vi "Reference Example.vi"() -> ()   [LabVIEW 2016, in "CS++Core-Examples.lvlib"]
doc: "This example illustrates how to use a factory to create a referenced initialized object and how to deal with it."
uses:
  CS++Core-Examples.lvlib
  CSPP_Core/Classes/CS++BaseClasses/Factory/CS++Factory.lvclass
  CSPP_Core/Classes/CS++BaseClasses/Factory/CS++Factory.lvclass/CS++Factory.ctl
  CSPP_Core/Classes/CS++BaseClasses/Reference/CS++Reference.lvclass/CS++Reference.ctl
  CSPP_Core/Classes/CS++BaseClasses/Factory/Write DB Connection String.vi
  CSPP_Core/Classes/CS++BaseClasses/Reference/CS++Reference.lvclass
  Classes/Example/Example.lvclass
panel:
  out "Error Out":errorcluster
  out "Object Name 2":string
  out "timed out?":bool
  out "Found?":bool
  out "timed out? 2":bool
  out "timed out? 1":bool
  in  "File Path Control":path=path "C:/User/Brand/Git/CSPP/Core/CS++Example.ini"
  in  "Object Name":string="myNumber"
  out "Number":dbl
  out "Attributes found?":bool
  out "Created new?":bool
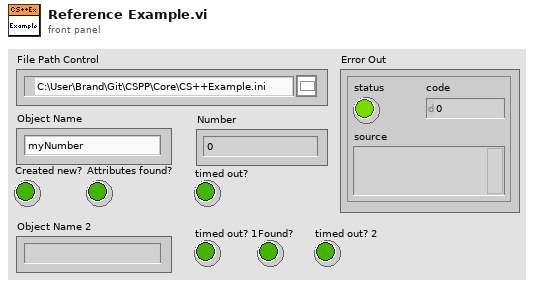
[diagram p1: front panel]
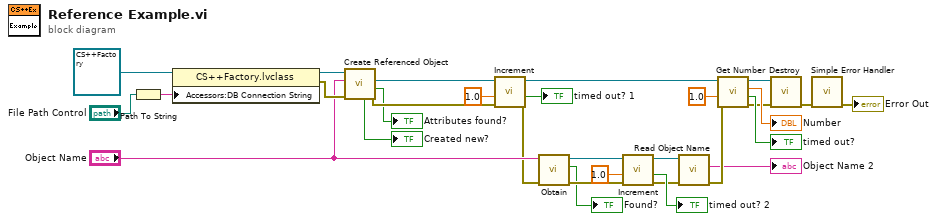
[diagram p0: block diagram]
diagram:
  n1 = Path To String(path="File Path Control") -> (string=w27:string)
  n2 = property class="CS++Factory.lvclass"(reference=refnum<class "CS++Factory.lvclass"> refnum ("CS++Factory in"), "Accessors:DB Connection String"=w27) -> (reference out=w29:refnum<class "CS++Factory.lvclass">, error out=w28:errorcluster)  [unwired: 1 in]
  n3 = call "Create Referenced Object.vi"("error in (no error)"=w28, "Object Name"="Object Name", "CS++Factory in"=w29) -> ("error out"=w23:errorcluster, "Attributes found?"=→"Attributes found?":bool, "CS++Base Reference"=w24:refnum<class "CS++Reference.lvclass">, "Created new?"=→"Created new?":bool)  [unwired: 4 in, 1 out]
  n4 = call "Increment.vi"("error in (no error)"=w23, "Timeout (-1)"=dbl[unit] 1.0, "Object Ref."=w24) -> ("error out"=w20:errorcluster, "timed out?"=→"timed out? 1":bool, "Object Ref. out"=w14:refnum<class "CS++Reference.lvclass">)  [unwired: 6 in]
  n5 = call "Obtain.vi"("Error In"=w20, "Object Name"="Object Name") -> ("Error Out"=w16:errorcluster, "Found?"=→"Found?":bool, "Object Reference"=w17:refnum<class "CS++Reference.lvclass">)  [unwired: 7 in]
  n6 = call "Increment.vi"("error in (no error)"=w16, "Timeout (-1)"=dbl[unit] 1.0, "Object Ref."=w17) -> ("error out"=w8:errorcluster, "timed out?"=→"timed out? 2":bool, "Object Ref. out"=w9:refnum<class "CS++Reference.lvclass">)  [unwired: 6 in]
  n7 = call "Read Object Name.vi"("error in (no error)"=w8, "CS++Reference in"=w9) -> ("error out"=w7:errorcluster, "Object Name"=→"Object Name 2":string)  [unwired: 7 in, 1 out]
  n8 = call "Get Number.vi"("error in (no error)"=w7, "Timeout (-1)"=dbl[unit] 1.0, "Object Ref."=w14) -> ("error out"=w4:errorcluster, "timed out?"=→"timed out?":bool, "Number"=→"Number":dbl, "Object Ref. out"=w13:refnum<class "CS++Reference.lvclass">)  [unwired: 5 in]
  n9 = call "Destroy.vi"("error in (no error)"=w4, "CS++Reference in"=w13) -> ("error out"=w5:errorcluster)  [unwired: 7 in, 2 out]
  n10 = call <vilib>:"Simple Error Handler.vi"("error in (no error)"=w5) -> ("error out"=→"Error Out":errorcluster)  [unwired: 4 in, 4 out]
